vi "Compound Arithmetic.vi"() -> ()   [LabVIEW 2020]
panel:
  out "result":dbl
  in  "Numeric 3":dbl
  in  "Numeric 2":dbl
  in  "Numeric":dbl
  # "Compound Arithmetic"
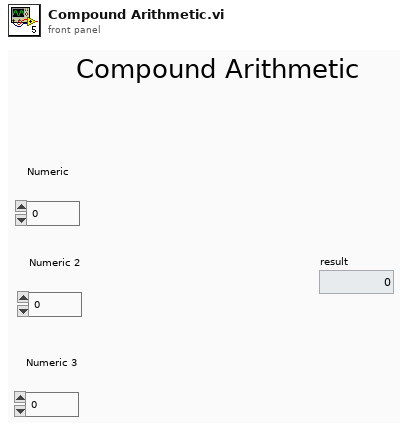
[diagram p1: front panel]
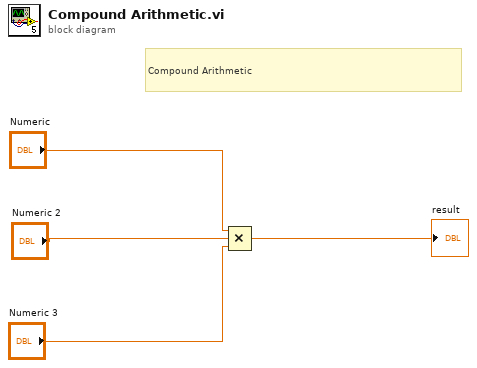
[diagram p0: block diagram]
diagram:
  # "Compound Arithmetic"
  n1 = Compound Arithmetic op=MULTIPLY("Numeric", "Numeric 2", "Numeric 3") -> (→"result":dbl)
